vi "SSH_Close.vi"(8 "error in (no error)":errorcluster, 11 "Python":T1) -> (0 "error out":errorcluster, 2 "return value":string)   [LabVIEW 2021]
uses:
  PythonCtrl.ctl
  Processors.ctl
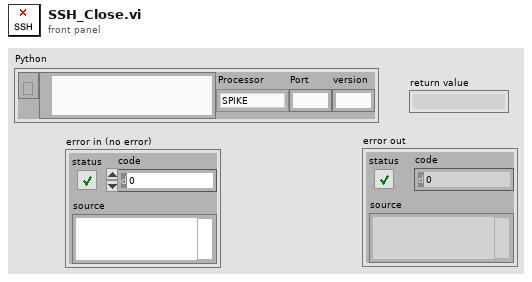
[diagram p1: front panel]
types:
  T1 = typedef "PythonCtrl.ctl" = cluster{"session":refnum<k35>, "PyPath":path, "Processor":T2, "Port":string, "version":string}
  T2 = typedef "Processors.ctl" = enum16{"SPIKE", "Pi", "Pi_ssh", "OpenMV", "Dunio"}
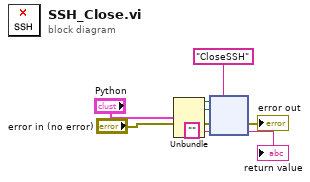
[diagram p0: block diagram]
diagram:
  n1 = Unbundle("Python") -> ("session"=w7:refnum<k35>, "PyPath"=w8:path)  [unwired: 3 out]
  n2 = node(w7, w8, "CloseSSH" ("function name"), "error in (no error)", "" ("function name")) -> (→"error out":errorcluster, →"return value":string)  [unwired: 3 out]
